vi "ChangeOverGui-DMCAccept.vi"(8 "error in":errorcluster, 10 "Configuration":i32) -> (0 "error out":errorcluster)   [LabVIEW 2016]
uses:
  ChangeOverGui.Action.ctl
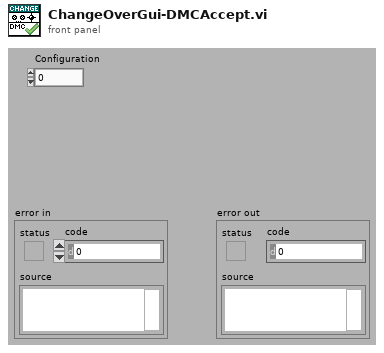
[diagram p1: front panel]
types:
  T1 = typedef "ChangeOverGui.Action.ctl" = enum32{"idle", "constructor", "destructor", "---ChangeOverGui ---", "Clear", "Validate", "Read File", "Read Imgs", "Check", "Accept", "Reject", "Scan.Begin", "Scan", "Update Table", "Update Counter", "DMC Accept"}
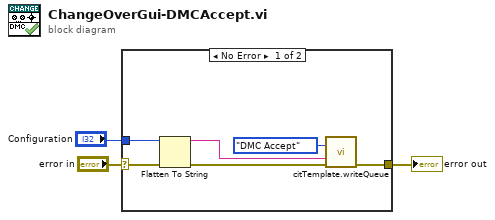
[diagram p0: block diagram]
diagram:
  n1 = case shown="No Error" "error in" {
    selector: "error in" -> [w9 w10]
    tunnel: [w7 w10] -> w2
    tunnel: "Configuration" -> [w4 _]
    frame No Error {
      n2 = Flatten To String(anything=w4, error in (no error)=w9) -> (data string=w5:string, error out=w6:errorcluster)  [unwired: 2 in, 1 out]
      n3 = call "citTemplate.writeQueue.vi"("event in (if not connected:all statemachine with data event)"=ChangeOverGui.Action."DMC Accept" ("Action"), "data in"=w5, "error in (no error)"=w6) -> ("error out"=w7:errorcluster)  [unwired: 12 in]
    }
    frame Error {
    }
  }
  "error out" <- w2
